vi "Write.vi"(8 "error in":errorcluster, 11 "Cluster.lvclass in":refnum<class "Cluster.lvclass">) -> (0 "error out":errorcluster, 3 "Cluster.lvclass out":refnum<class "Cluster.lvclass">)   [LabVIEW 2023, in "Cluster.lvclass"]
uses:
  Cluster.lvclass
  Cluster.lvclass/Cluster.ctl
  6bfc6677-cd67-4f2d-afef-839dec9218ce.vi
  74f11eb1-9425-41af-a169-6608e4aa6674.vi
  6bfc6677-cd67-4f2d-afef-839dec9218ce.vi/4bc1c15b-36ab-481f-b8dd-c64075ce723a.vi
  6bfc6677-cd67-4f2d-afef-839dec9218ce.vi/d83cb72b-7713-41fc-a3d1-682de79cf574.vi
  74f11eb1-9425-41af-a169-6608e4aa6674.vi/4bc1c15b-36ab-481f-b8dd-c64075ce723a.vi
  74f11eb1-9425-41af-a169-6608e4aa6674.vi/d83cb72b-7713-41fc-a3d1-682de79cf574.vi
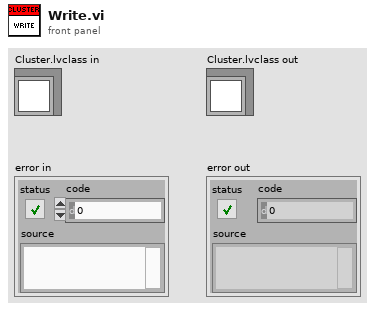
[diagram p1: front panel]
types:
  T1 = typedef "Cluster.lvclass/Producer Control.ctl" = cluster{"OnOff.STS":i32, "Error.STS":i32, "Watchdog.STS":i32}
  T2 = typedef "Cluster.lvclass/Producer Ch.ctl" = cluster{"OutputEnable.STS":i32, "ControlMode.STS":u16, "Actual Value.AV":dbl}
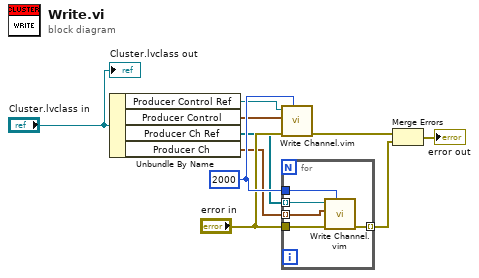
[diagram p0: block diagram]
diagram:
  w10 = 2000 ("Timeout (ms)")
  n1 = Unbundle By Name("Cluster.lvclass in") -> ("Producer Control Ref"=w9:refnum<k21>, "Producer Control"=w3:T1, "Producer Ch Ref"=w2:refnum<k21>[], "Producer Ch"=w1:T2[])
  n2 = call "Write Channel.vim"("Timeout (ms)"=w10, "error in"="error in", "Data in"=w3, "ADAS HIL Channel in"=w9) -> ("error out"=w7:errorcluster)  [unwired: 5 in, 2 out]
  n3 = for {
    tunnel: "error in" -> [w15]
    tunnel: [w14] -> w6 mode=indexing
    tunnel: w2 -> [w13] mode=indexing
    tunnel: w10 -> [w12]
    tunnel: w1 -> [w11] mode=indexing
    n4 = call "Write Channel.vim"("Timeout (ms)"=w12, "error in"=w15, "Data in"=w11, "ADAS HIL Channel in"=w13) -> ("error out"=w14:errorcluster)  [unwired: 5 in, 2 out]
  }
  n5 = Merge Errors(w7, w6) -> (→"error out":errorcluster)
  "Cluster.lvclass out" <- "Cluster.lvclass in"
